vi "DHT11_labview_srednia_symulacja.vi"() -> ()   [LabVIEW 2025]
uses:
  <vilib>/Utility/error.llb/Trim Whitespace One-Sided.vi
panel:
  out "Temperatura œrednia[C]":dbl
  out "Wilgotnoœæ œrednia[%]":dbl
  out "Temperatura min[C]":dbl
  out "Temperatura max [C]":dbl
  out "Wilogtnoœæ min [%]":dbl
  out "Wilgotnosc max [%]":dbl
  out "Numeric":i32
  out "wilgotnoœæ liczba":dbl
  out "Wilgotnoœæ wykres":dbl(graph)
  out "Temperatura liczba":dbl
  out "Temperatura wykres":dbl(graph)
  out "wyœwietlanie danych":string
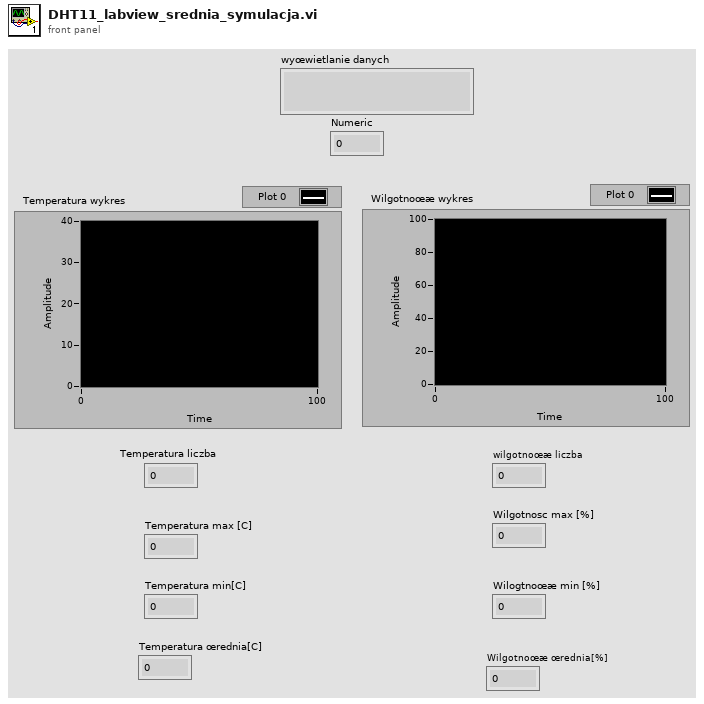
[diagram p1: front panel]
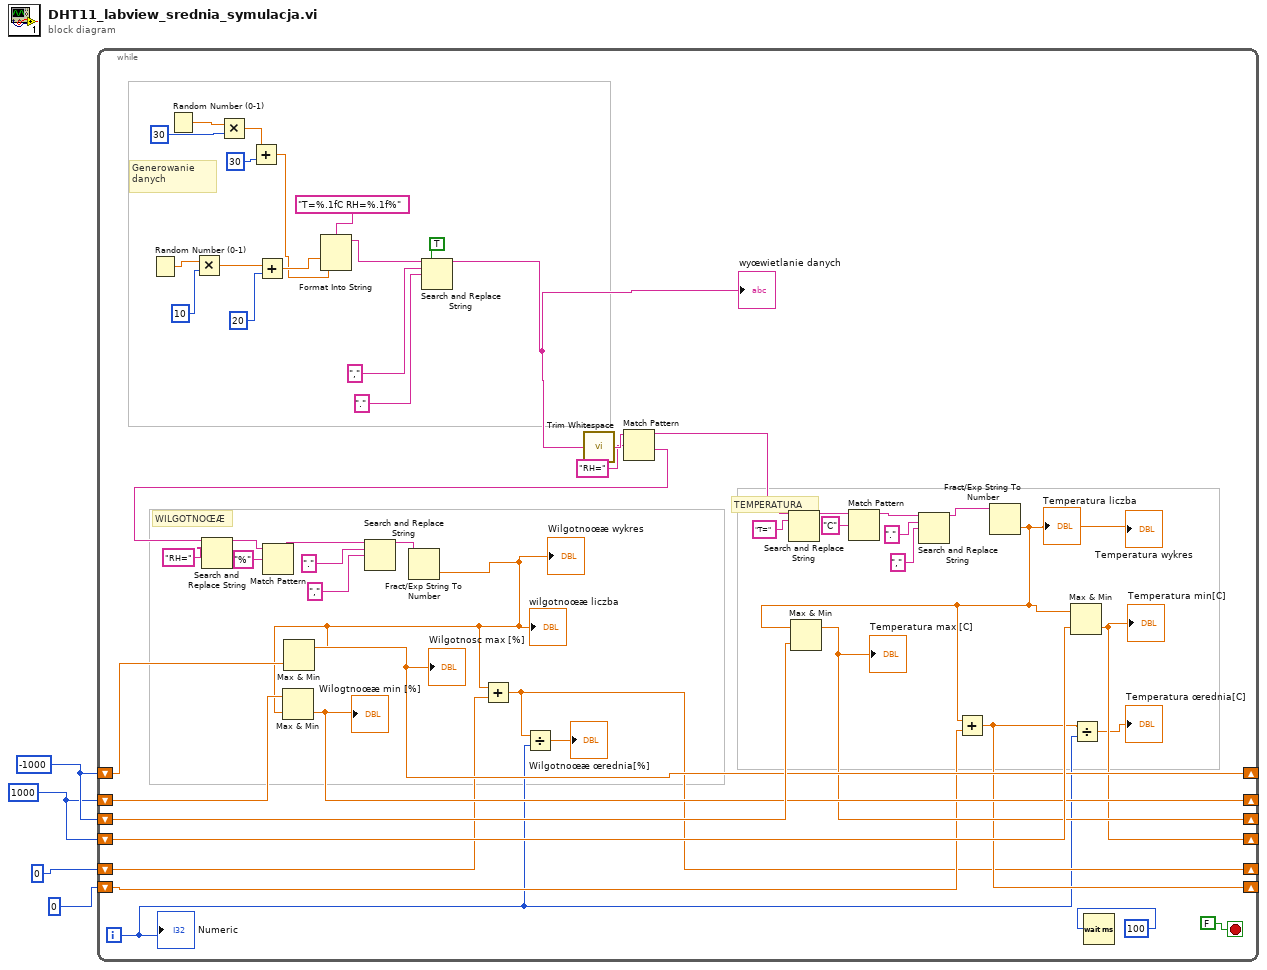
[diagram p0: block diagram]
diagram:
  w3 = 1000
  w4 = -1000
  n1 = while {
    shift-right: [w17] -> _
    shift-left: w4 -> [w21]
    shift-right: [w16] -> _
    shift-left: w3 -> [w20]
    shift-right: [w15] -> _
    shift-left: w4 -> [w19]
    shift-right: [w14] -> _
    shift-left: w3 -> [w18]
    shift-right: [w6] -> _
    shift-left: 0 -> [w13]
    shift-right: [w8] -> _
    shift-left: 0 -> [w10]
    i -> [w5]
    stop <- FALSE stop-if-true
    # "Generowanie danych"
    # "WILGOTNOŒÆ"
    # "TEMPERATURA"
    n2 = Random Number (0-1)() -> (number: 0 to 1=w34:dbl)
    n3 = Random Number (0-1)() -> (number: 0 to 1=w36:dbl)
    n4 = Multiply(x=w34, y=10) -> (x*y=w35:dbl)
    n5 = Multiply(x=w36, y=30) -> (x*y=w37:dbl)
    n6 = Add(x=w37, y=30) -> (x+y=w22:dbl)
    n7 = Add(x=w35, y=20) -> (x+y=w23:dbl)
    n8 = Format Into String(format string="T=%.1fC RH=%.1f%", w23, w22) -> (resulting string=w24:string)  [unwired: 2 in, 1 out]
    n9 = Search and Replace String(replace all?=TRUE, input string=w24, search string=",", replace string=".") -> (result string=w26:string)  [unwired: 4 in, 3 out]
    "wyœwietlanie danych" <- w26
    n10 = call <vilib>:"Trim Whitespace.vi"("string"=w26) -> ("trimmed string"=w48:string)  [unwired: 1 in]
    n11 = Match Pattern(string=w48, regular expression="RH=") -> (before substring=w49:string, after substring=w53:string)  [unwired: 1 in, 2 out]
    n12 = Search and Replace String(input string=w53, search string="RH=") -> (result string=w54:string)  [unwired: 6 in, 3 out]
    n13 = Match Pattern(string=w54, regular expression="%") -> (before substring=w55:string)  [unwired: 1 in, 3 out]
    n14 = Search and Replace String(input string=w55, search string=".", replace string="," ("replace string (\"\")")) -> (result string=w56:string)  [unwired: 5 in, 3 out]
    n15 = Fract/Exp String To Number(string=w56) -> (number=w12:dbl)  [unwired: 3 in, 1 out]
    "Wilgotnoœæ wykres" <- w12
    "wilgotnoœæ liczba" <- w12
    n16 = Max & Min(x=w20, y=w12) -> (min(x,y)=w16:dbl)  [unwired: 1 out]
    "Wilogtnoœæ min [%]" <- w16
    n17 = Max & Min(x=w12, y=w21) -> (max(x,y)=w17:dbl)  [unwired: 1 out]
    "Wilgotnosc max [%]" <- w17
    n18 = Add(x=w12, y=w13) -> (x+y=w6:dbl)
    n19 = Divide(x=w6, y=w5) -> (x/y=→"Wilgotnoœæ œrednia[%]":dbl)
    n20 = Search and Replace String(input string=w49, search string="T=" ("replace string (\"\")")) -> (result string=w50:string)  [unwired: 6 in, 3 out]
    n21 = Match Pattern(string=w50, regular expression="C") -> (before substring=w51:string)  [unwired: 1 in, 3 out]
    n22 = Search and Replace String(input string=w51, search string=".", replace string="," ("replace string (\"\")")) -> (result string=w52:string)  [unwired: 5 in, 3 out]
    n23 = Fract/Exp String To Number(string=w52) -> (number=w11:dbl)  [unwired: 3 in, 1 out]
    "Temperatura wykres" <- w11
    "Temperatura liczba" <- w11
    n24 = Max & Min(x=w11, y=w19) -> (max(x,y)=w15:dbl)  [unwired: 1 out]
    "Temperatura max [C]" <- w15
    n25 = Add(x=w11, y=w10) -> (x+y=w8:dbl)
    n26 = Max & Min(x=w11, y=w18) -> (min(x,y)=w14:dbl)  [unwired: 1 out]
    "Temperatura min[C]" <- w14
    n27 = Divide(x=w8, y=w5) -> (x/y=→"Temperatura œrednia[C]":dbl)
    n28 = Wait (ms)(milliseconds to wait=u32 100) -> ()  [unwired: 1 out]
    "Numeric" <- w5
  }
